vi "DateTime.vi"() -> (3 "DateTime":string)   [LabVIEW 2018]
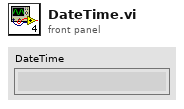
[diagram p1: front panel]
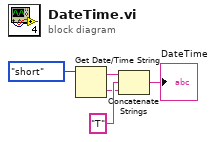
[diagram p0: block diagram]
diagram:
  n1 = Get Date/Time String(date format (0)=enum16{"short", "long", "abbreviated"}."short" ("日期格式(0)")) -> (date string=w3:string, time string=w2:string)  [unwired: 2 in]
  n2 = Concatenate Strings(w3, "T" ("字符串"), w2) -> (→"DateTime":string)
